vi "GetFilePaths.vi"(8 "error in (no error)":errorcluster) -> (0 "error out":errorcluster, 2 "FilePaths out":path[](array[path]))   [LabVIEW 2017]
doc: "returns all available file-paths from the source folder (given in global variable)"
uses:
  global_variables.vi
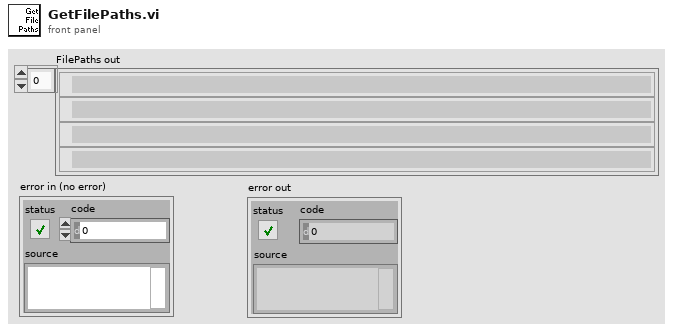
[diagram p1: front panel]
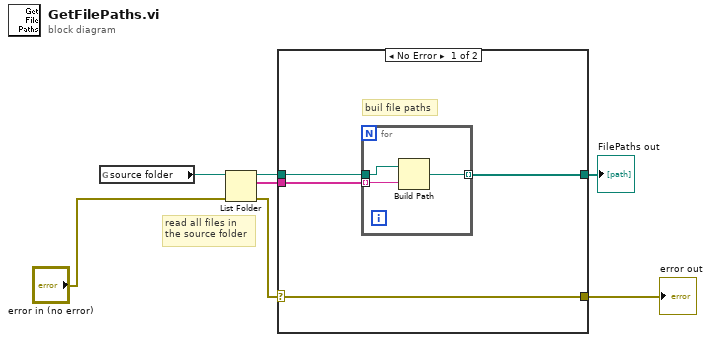
[diagram p0: block diagram]
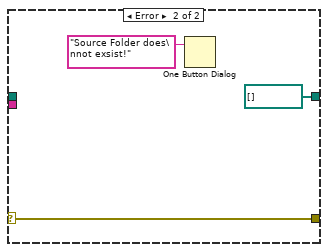
[diagram p2: hidden frame]
diagram:
  # "read all files in\nthe source folder"
  n1 = global read "global_variables.vi" "source folder"() -> (w7:path)
  n2 = List Folder(path=w7, error in="error in (no error)") -> (path out=w5:path, filenames=w4:string[], error out=w6:errorcluster)  [unwired: 2 in, 1 out]
  n3 = case shown="No Error" w6 {
    selector: w6 -> [w10 w16]
    tunnel: w5 -> [w9 _]
    tunnel: w4 -> [w11 _]
    tunnel: [w10 w16] -> w2
    tunnel: [w8 path[] []] -> w1
    frame No Error {
      # "buil file paths"
      n4 = for {
        tunnel: w11 -> [w13] mode=indexing
        tunnel: w9 -> [w14]
        tunnel: [w12] -> w8 mode=indexing
        n5 = Build Path(base path=w14, name or relative path=w13) -> (appended path=w12:path)
      }
    }
    frame Error {
      n6 = One Button Dialog(message="Source Folder does\nnot exsist!") -> ()  [unwired: 1 in, 1 out]
    }
  }
  "error out" <- w2
  "FilePaths out" <- w1
